vi "Configure Datum.vi"(0 "VISA resource name":refnum<visa-resource-name>, 5 "Datum (Standard)":u16(ring)=1 items=["Standard (WGS84)", "User Defined"], 7 "User defined datum":i8[](array[numeric])=[0, 1, 0, 0], 9 "Timeout (1000 ms)":u32=1000, 11 "error in (no error)":errorcluster) -> (4 "VISA resource name out":refnum<visa-resource-name>, 6 "Configure Datum Successful":bool, 15 "error out":errorcluster)   [LabVIEW 2009]
doc: "Allows the user to configure the device for the standard datum, or specify another datum."
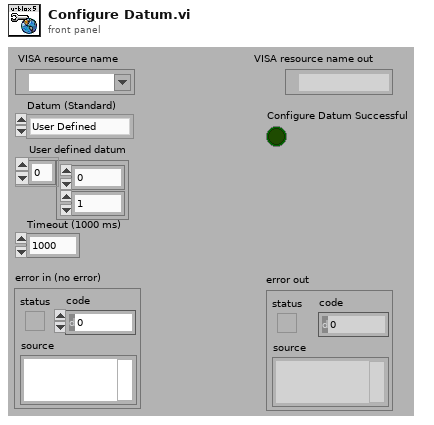
[diagram p1: front panel]
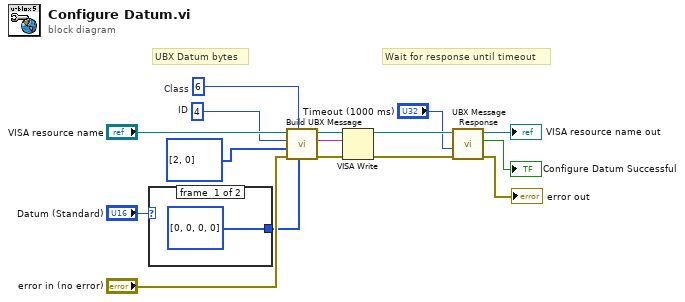
[diagram p0: block diagram]
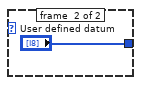
[diagram p2: hidden frame]
diagram:
  w1 = i8 4  # ID
  w9 = i8 6  # Class
  # "UBX Datum bytes"
  # "Wait for response until timeout"
  n1 = case shown="0, Default" "Datum (Standard)" {
    tunnel: [i8[] [0, 0, 0, 0] "User defined datum"] -> w7
    frame #0 {
    }
    frame #1 {
    }
  }
  n2 = call "Build UBX Message.vi"("Payload"=w7, "Class"=w9, "error in"="error in (no error)", "Length"=i8[] [2, 0], "ID"=w1, "VISA resource name"="VISA resource name") -> ("error out"=w5:errorcluster, "UBX Message"=w4:string, "VISA resource name out"=w3:refnum<visa-resource-name>)  [unwired: 3 out]
  n3 = VISA Write(VISA resource name=w3, write buffer=w4, error in (no error)=w5) -> (VISA resource name out=w16:refnum<visa-resource-name>, error out=w15:errorcluster)  [unwired: 1 out]
  n4 = call "UBX Message Response.vi"("error in"=w15, "Timeout (1000 ms)"="Timeout (1000 ms)", "VISA resource name"=w16) -> ("error out"=→"error out":errorcluster, "Message Acknowledged"=→"Configure Datum Successful":bool, "VISA resource name out"=→"VISA resource name out":refnum<visa-resource-name>)  [unwired: 1 in, 5 out]
